vi "Calibrate.vi"(8 "error in (no error)":errorcluster, 11 "EXFO in":refnum<class "EXFO.lvclass">) -> (0 "error out":errorcluster, 3 "EXFO out":refnum<class "EXFO.lvclass">)   [LabVIEW 2018, in "EXFO.lvlib" / "EXFO.lvclass"]
doc: "This is a parent VI. The children VI will overwrite this with the correct calls for calibration.\n\nAuthor: Ron Dexter\nCompany: Luminar\nModified: 5/20/2018"
uses:
  EXFO.lvclass
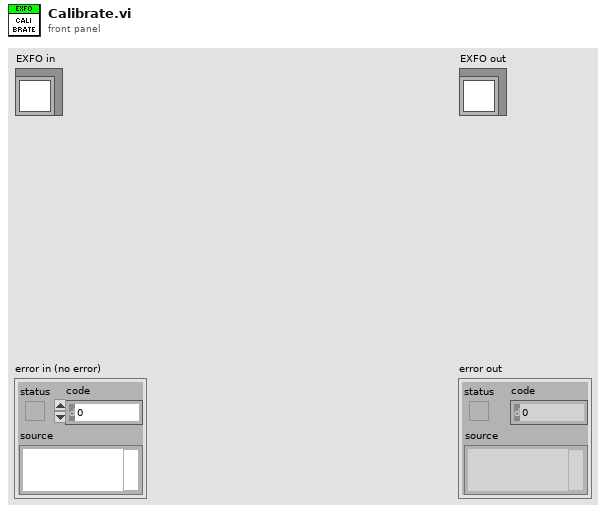
[diagram p1: front panel]
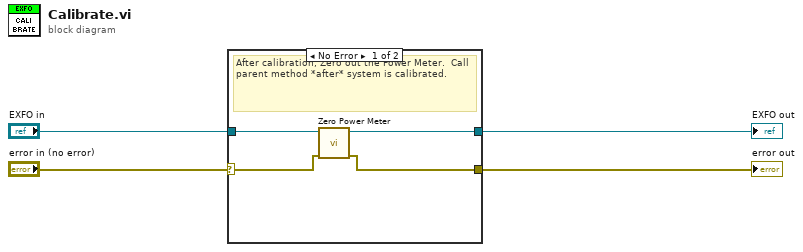
[diagram p0: block diagram]
diagram:
  n1 = case shown="No Error" "error in (no error)" {
    selector: "error in (no error)" -> [w6 w10]
    tunnel: [w5 w10] -> w3
    tunnel: [w7 w9] -> w1
    tunnel: "EXFO in" -> [w8 w9]
    frame No Error {
      # "After calibration, Zero out the Power Meter.  Call parent method *after* system is calibrated."
      n2 = call-dynamic "Zero Power Meter.vi"("error in (no error)"=w6, "EXFO in"=w8) -> ("error out"=w5:errorcluster, "EXFO out"=w7:refnum<class "EXFO.lvclass">)  [unwired: 8 in]
    }
    frame Error {
    }
  }
  "error out" <- w3
  "EXFO out" <- w1
